vi "Logger2.vi"() -> (3 "Log out":string)   [LabVIEW 2023]
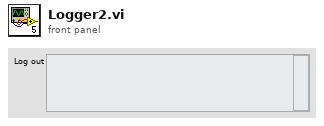
[diagram p1: front panel]
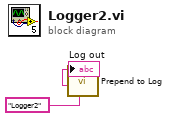
[diagram p0: block diagram]
diagram:
  n1 = call "Prepend to Log.vi"("new entry"="Logger2") -> ("Log out"=→"Log out":string)  [unwired: 10 in]
